vi "Run Bfr Rx - CachedSize - Copy Flush Add.vi"(4 "Data Size in":u64, 6 "Copy and Flush":bool, 7 "External Buffer":u64 format="%016x", 8 "error in (no error)":errorcluster, 10 "Data in":u8[](array[numeric]), 11 "Cached Buffer in":T1 {"Cache Buffer" format="%016x"}) -> (0 "error out":errorcluster, 3 "Cached Buffer out":T1 {"Cache Buffer" format="%016x"})   [LabVIEW 2016, in "UDP-Custom-Device Engine.lvlib"]
uses:
  UDP-Custom-Device Engine.lvlib
  Types/Engine - Buffered Rx Cached Buffer.ctl
  <vilib>/NI Veristand/VeriStand Data/Pointer Operations/Pointer.In-Place Read.vi
  <vilib>/NI Veristand/VeriStand Data/Pointer Operations/Pointer.In-Place Read (1D U8).vi
  <vilib>/NI Veristand/VeriStand Data/Pointer Operations/Pointer.Write.vi
  <vilib>/NI Veristand/VeriStand Data/Pointer Operations/Pointer.Write (1D U8).vi
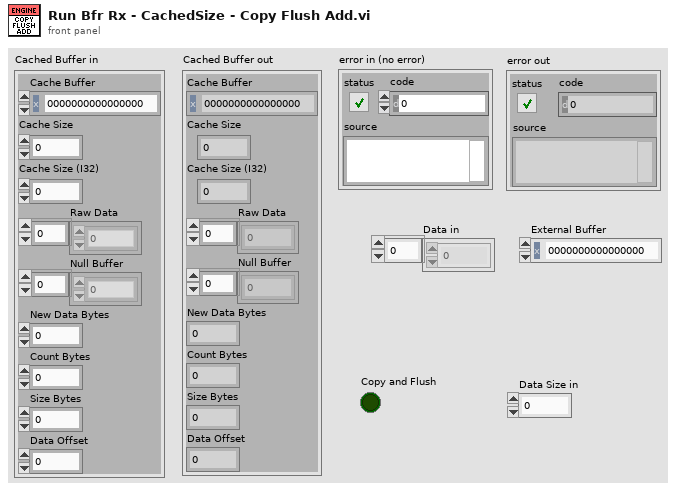
[diagram p1: front panel]
types:
  T1 = typedef "UDP-Custom-Device Engine.lvlib/Engine - Buffered Rx Cached Buffer.ctl" = cluster{"Cache Buffer":u64, "Cache Size":u64, "Cache Size (I32)":i32, "Raw Data":u8[], "Null Buffer":u8[], "New Data Bytes":u64, "Count Bytes":u64, "Size Bytes":u64, "Data Offset":u64}
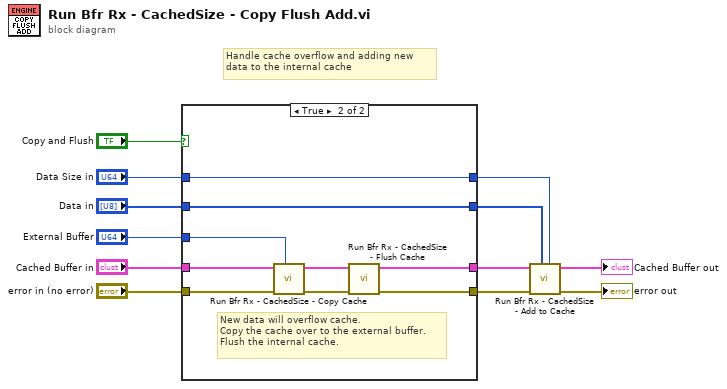
[diagram p0: block diagram]
diagram:
  # "Handle cache overflow and adding new\ndata to the internal cache"
  n1 = case shown="True" "Copy and Flush" {
    tunnel: [w15 w21] -> w5
    tunnel: "Cached Buffer in" -> [w15 w25]
    tunnel: [w16 w19] -> w3
    tunnel: "error in (no error)" -> [w16 w24]
    tunnel: "External Buffer" -> [_ w23]
    tunnel: "Data in" -> [w14 w18]
    tunnel: "Data Size in" -> [w13 w17]
    tunnel: [w14 w18] -> w2
    tunnel: [w13 w17] -> w1
    frame False {
      # "There is still space in the cache for more\ndata. Skip copy/flush and add the new\ndata to the cache."
    }
    frame True {
      # "New data will overflow cache.\nCopy the cache over to the external buffer.\nFlush the internal cache."
      n2 = call "Run Bfr Rx - CachedSize - Copy Cache.vi"("External Buffer"=w23, "error in (no error)"=w24, "Cached Buffer in"=w25) -> ("error out"=w20:errorcluster, "Cached Buffer out"=w22:T1)  [unwired: 7 in]
      n3 = call "Run Bfr Rx - CachedSize - Flush Cache.vi"("error in (no error)"=w20, "Cached Buffer in"=w22) -> ("error out"=w19:errorcluster, "Cached Buffer out"=w21:T1)  [unwired: 8 in]
    }
  }
  n4 = call "Run Bfr Rx - CachedSize - Add to Cache.vi"("Data Size in"=w1, "Data in"=w2, "error in (no error)"=w3, "Cached Buffer in"=w5) -> ("error out"=→"error out":errorcluster, "Cached Buffer out"=→"Cached Buffer out":T1)  [unwired: 6 in]
